vi "Read Error Handling Parameters.vi"(4 "Error In":errorcluster, 7 "Config Data in":refnum<class "Config Data.lvclass">) -> (0 "Error Out":errorcluster, 1 "Buttons":T1={"Continue/Ok Button"="Continue", "Stop Button"="Stop"}, 2 "Action":T2(ring), 3 "Config Data out":refnum<class "Config Data.lvclass">)   [LabVIEW 2014, in "Config Data.lvlib" / "Config Data.lvclass"]
uses:
  Config Data.lvclass
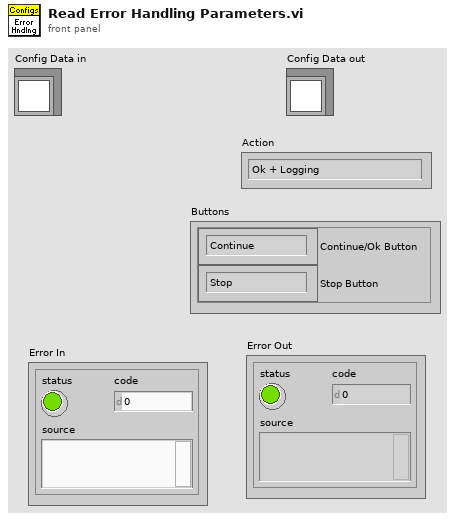
[diagram p1: front panel]
types:
  T1 = cluster{"Continue/Ok Button":string, "Stop Button":string}
  T2 = enum16{"Ok + Logging", "Continue/Stop + Logging", "Logging Only", "Ok Only", "Continue/Stop Only"}
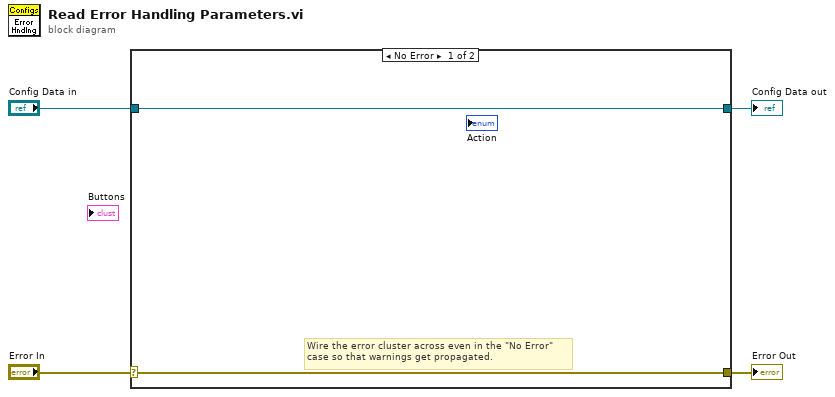
[diagram p0: block diagram]
diagram:
  n1 = case shown="No Error" "Error In" {
    selector: "Error In" -> [w5 w8]
    tunnel: [w5 w8] -> w3
    tunnel: [w6 w7] -> w1
    tunnel: "Config Data in" -> [w6 w7]
    frame No Error {
      # "Wire the error cluster across even in the \"No Error\"\ncase so that warnings get propagated."
    }
    frame Error {
    }
  }
  "Error Out" <- w3
  "Config Data out" <- w1
